vi "LoadMotors.vi"(8 "error in (no error)":errorcluster, 11 "MotorController in":refnum<class "MotorController.lvclass">) -> (0 "error out":errorcluster, 3 "MotorController out":refnum<class "MotorController.lvclass">)   [LabVIEW 2019, in "MotorController.lvclass"]
uses:
  MotorController.lvclass
  MotorController.lvclass/MotorController.ctl
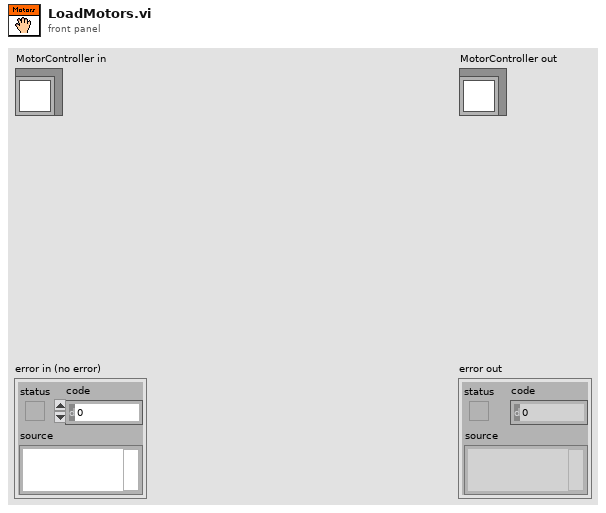
[diagram p1: front panel]
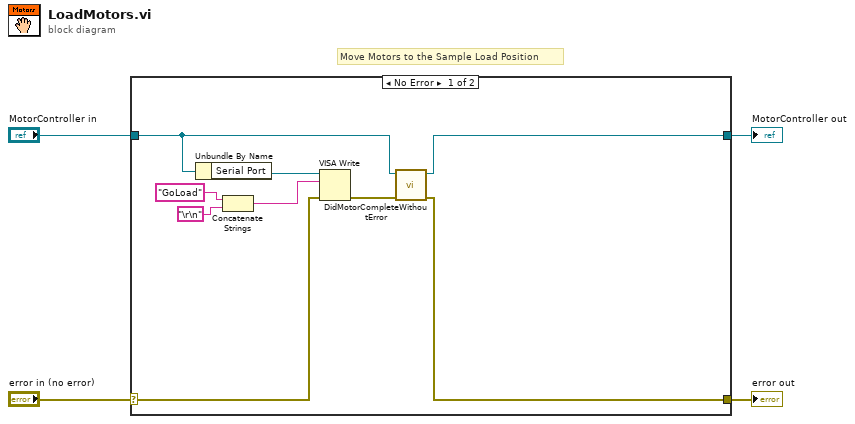
[diagram p0: block diagram]
diagram:
  # "Move Motors to the Sample Load Position"
  n1 = case shown="No Error" "error in (no error)" {
    selector: "error in (no error)" -> [w9 w15]
    tunnel: [w5 w15] -> w3
    tunnel: [w7 w14] -> w1
    tunnel: "MotorController in" -> [w8 w14]
    frame No Error {
      n2 = Unbundle By Name(w8) -> ("Serial Port"=w13:refnum<visa-resource-name>)
      n3 = Concatenate Strings("GoLoad", "\r\n") -> (w10:string)
      n4 = VISA Write(VISA resource name=w13, write buffer=w10, error in (no error)=w9) -> (error out=w6:errorcluster)  [unwired: 2 out]
      n5 = call "DidMotorCompleteWithoutError.vi"("error in (no error)"=w6, "MotorController in"=w8) -> ("error out"=w5:errorcluster, "MotorController out"=w7:refnum<class "MotorController.lvclass">)  [unwired: 7 in, 1 out]
    }
    frame Error {
    }
  }
  "error out" <- w3
  "MotorController out" <- w1
